vi "Wait For.vi"   [LabVIEW 2017, in "DSF Core.lvlib" / "Logging Interface.lvclass"]
uses:
  Logging Interface.lvclass
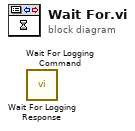
[diagram p0: block diagram]
diagram:
  n1 = call "Wait For Logging Response.vi"() -> ()  [unwired: 8 in, 4 out]
  n2 = call "Wait For Logging Command.vi"() -> ()  [unwired: 8 in, 4 out]
